vi "Complex Number to String (CDB 1D Array).vi"(1 "use system decimal point (T)":bool=TRUE, 2 "precision (6)":i16, 3 "width (-)":i16, 4 "number[]":cdb[](array[numeric])) -> (0 "Complex-format string []":string[](array[string]))   [LabVIEW 2018, in "Numeric Data Type.lvclass"]
doc: "<b> </b> <b> </b>\n©2013, Q Software Innovations, LLC.\n\nWritten in National Instruments LabVIEW™ 2013.\n\nAuthored by Quentin Alldredge\nQ@qsoftwareinnovations.com\nwww.qsoftwareinnovations.com\n\nAll rights reserved."
uses:
  Numeric Data Type.lvclass
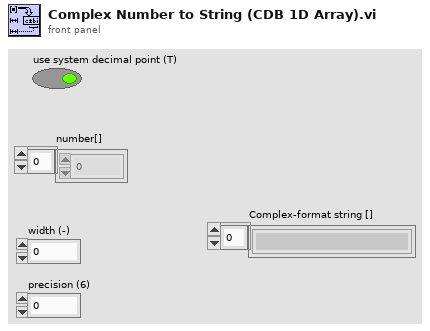
[diagram p1: front panel]
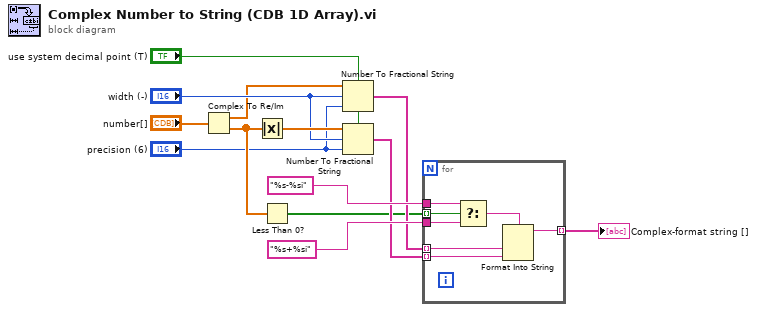
[diagram p0: block diagram]
diagram:
  n1 = Complex To Re/Im(x + iy="number[]") -> (x=w6:dbl[], y=w13:dbl[])
  n2 = Absolute Value(x=w13) -> (abs(x)=w12:dbl[])
  n3 = Less Than 0?(x=w13) -> (x < 0?=w1:bool[])
  n4 = Number To Fractional String(use system decimal point (T)="use system decimal point (T)", number=w6, width (-)="width (-)", precision (6)="precision (6)") -> (F-format string=w3:string[])
  n5 = Number To Fractional String(use system decimal point (T)="use system decimal point (T)", number=w12, width (-)="width (-)", precision (6)="precision (6)") -> (F-format string=w2:string[])
  n6 = for {
    tunnel: [w20] -> w7 mode=indexing
    tunnel: w1 -> [w19] mode=indexing
    tunnel: "%s+%si" -> [w18]
    tunnel: "%s-%si" -> [w17]
    tunnel: w3 -> [w15] mode=indexing
    tunnel: w2 -> [w14] mode=indexing
    n7 = Select(t=w17, s=w19, f=w18) -> (s? t:f=w16:string)
    n8 = Format Into String(format string=w16, w15, w14) -> (resulting string=w20:string)  [unwired: 2 in, 1 out]
  }
  "Complex-format string []" <- w7
